vi "PPMS field.vi"(2 "error in (no error)":errorcluster, 3 "Transmit Mode (0)":T1(ring), 4 "GPIB address":string="15") -> (0 "error out":errorcluster, 1 "Field (Oe)":dbl format="%.3f")   [LabVIEW 2018]
doc: "This returns the field in the sample chamber as reported by the PPMS system. Note that this is not the exact field, only that calculated from the current through the magnet."
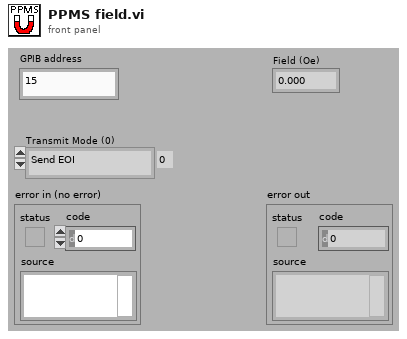
[diagram p1: front panel]
types:
  T1 = enum16{"Send EOI", "append CR w/ EOI", "append LF w/ EOI", "append CR LF w/ EOI", "append CR w/o EOI", "append LF w/o EOI", "append CR LF w/o EOI", "do not send EOI"}
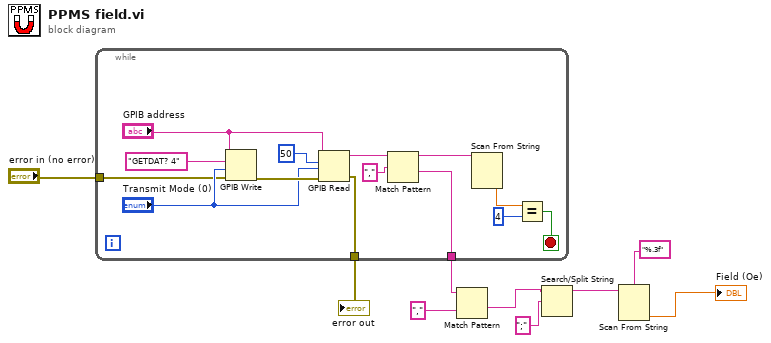
[diagram p0: block diagram]
diagram:
  n1 = while {
    tunnel: [w12] -> w6
    tunnel: [w11] -> w2
    tunnel: "error in (no error)" -> [w10]
    stop <- w13 stop-if-true
    n2 = GPIB Write(0:"GPIB address", 1:"GETDAT? 4", 2:"Transmit Mode (0)", 3:w10) -> (6:w22:errorcluster)  [unwired: 1 in, 1 out]
    n3 = GPIB Read(0:"GPIB address", 1:50, 2:"Transmit Mode (0)", 3:w22) -> (5:w17:string, 7:w11:errorcluster)  [unwired: 1 in, 1 out]
    n4 = Match Pattern(string=w17, regular expression=",") -> (before substring=w16:string, after substring=w12:string)  [unwired: 1 in, 2 out]
    n5 = Scan From String(input string=w16) -> (output 1=w15:dbl)  [unwired: 4 in, 3 out]
    n6 = Equal?(x=w15, y=4) -> (x = y?=w13:bool)
  }
  "error out" <- w2
  n7 = Match Pattern(string=w6, regular expression=",") -> (after substring=w4:string)  [unwired: 1 in, 3 out]
  n8 = Search/Split String(string=w4, search string/char (-)=";") -> (substring before match=w5:string)  [unwired: 1 in, 2 out]
  n9 = Scan From String(format string="%.3f", input string=w5) -> (output 1=→"Field (Oe)":dbl)  [unwired: 3 in, 3 out]
